vi "SortPoints.vi"(9 "Nominal Points":T2(array[cluster]), 10 "Actual Points":T2(array[cluster])) -> (1 "Nominal PointsOut":T2(array[cluster]), 2 "Actual Points Out":T2(array[cluster]))   [LabVIEW 2017]
uses:
  AT901 API/Structures/Struct TransformationPoint.ctl
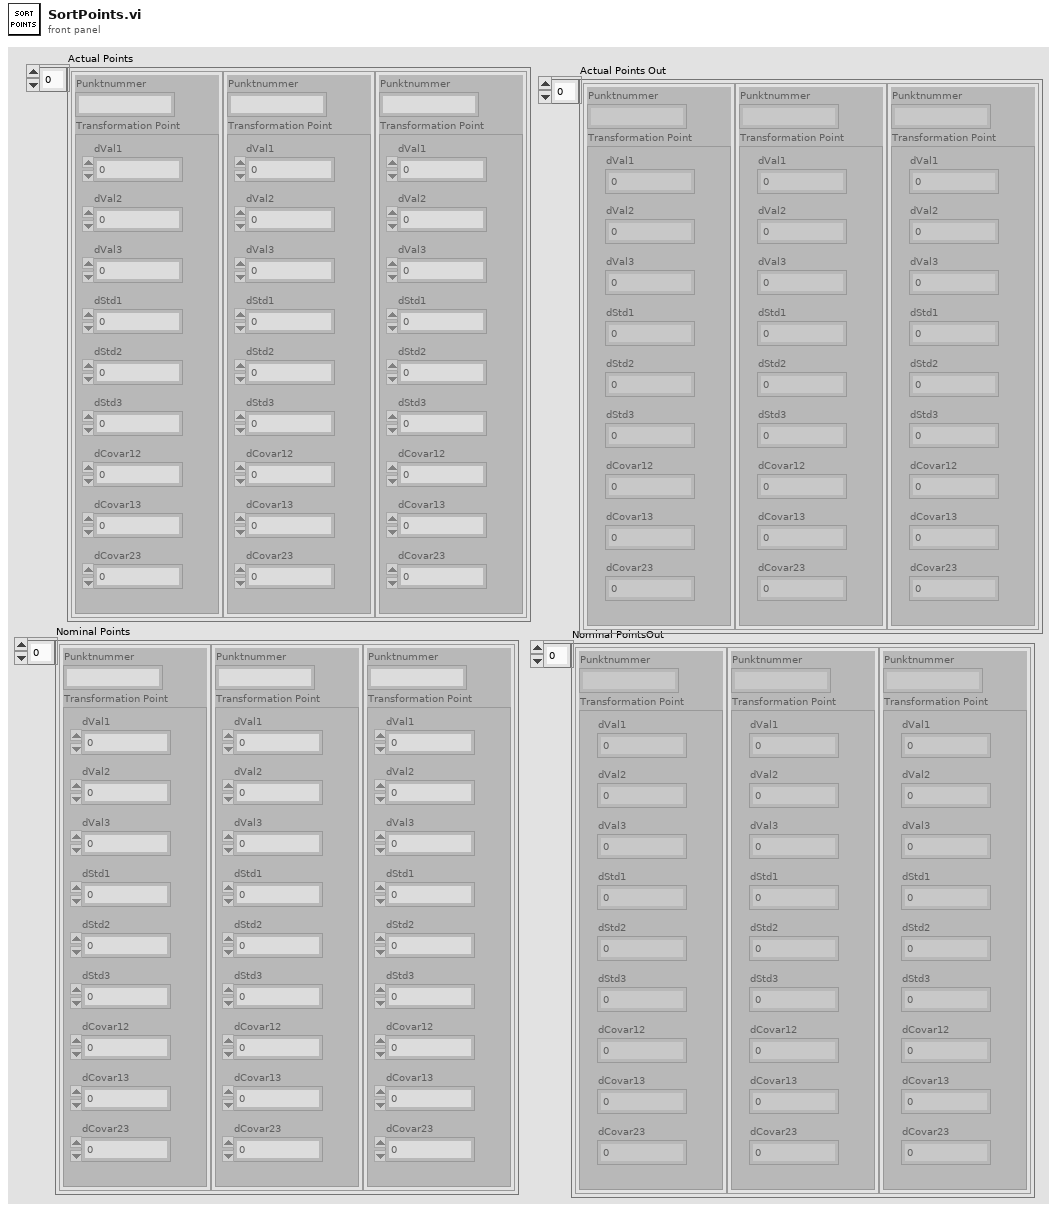
[diagram p1: front panel]
types:
  T1 = typedef "Struct TransformationPoint.ctl" = cluster{"dVal1":dbl, "dVal2":dbl, "dVal3":dbl, "dStd1":dbl, "dStd2":dbl, "dStd3":dbl, "dCovar12":dbl, "dCovar13":dbl, "dCovar23":dbl}
  T2 = cluster{"Punktnummer":string, "Transformation Point":T1}[]
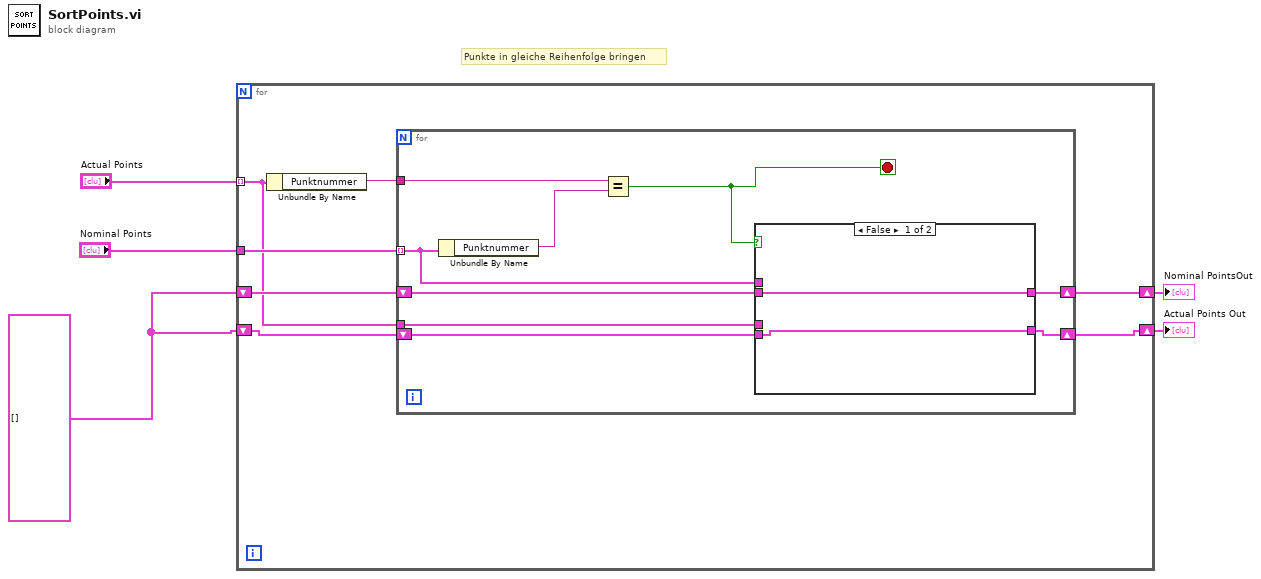
[diagram p0: block diagram]
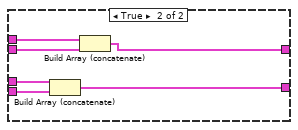
[diagram p2: hidden frame]
diagram:
  w3 = T2 []
  # "Punkte in gleiche Reihenfolge bringen"
  n1 = for {
    tunnel: "Actual Points" -> [w8] mode=indexing
    tunnel: "Nominal Points" -> [w12]
    shift-right: [w10] -> w2
    shift-left: w3 -> [w9]
    shift-right: [w7] -> w1
    shift-left: w3 -> [w6]
    n2 = Unbundle By Name(w8) -> ("Punktnummer"=w11:string)
    n3 = for {
      tunnel: w12 -> [w18] mode=indexing
      tunnel: w11 -> [w21]
      shift-right: [w17] -> w10
      shift-left: w9 -> [w16]
      tunnel: w8 -> [w15]
      shift-right: [w14] -> w7
      shift-left: w6 -> [w13]
      stop <- w19 stop-if-true
      n4 = Unbundle By Name(w18) -> ("Punktnummer"=w20:string)
      n5 = Equal?(x=w21, y=w20) -> (x = y?=w19:bool)
      n6 = case shown="False" w19 {
        tunnel: w18 -> [_ w29]
        tunnel: [w23 w28] -> w17
        tunnel: w16 -> [w23 w27]
        tunnel: w15 -> [_ w26]
        tunnel: [w22 w25] -> w14
        tunnel: w13 -> [w22 w24]
        frame False {
        }
        frame True {
          n7 = Build Array (concatenate)(w26, w24) -> (w25:T2)
          n8 = Build Array (concatenate)(w29, w27) -> (w28:T2)
        }
      }
    }
  }
  "Nominal PointsOut" <- w2
  "Actual Points Out" <- w1
